vi "DNET Input.vi"(8 "stop":bool) -> (3 "DNET1":u32[](array[numeric]))   [LabVIEW 2011]
panel:
  in  "Slot":T1(ring)=enum."Dnet1"
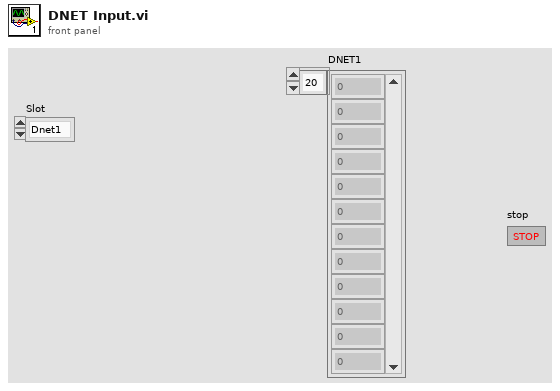
[diagram p1: front panel]
types:
  T1 = enum16{"NC1", "NC2", "Dnet1", "Dnet2", "Dnet3", "Ain1", "Ain2", "Aout1", "Din1", "Din2", "Dout1"}
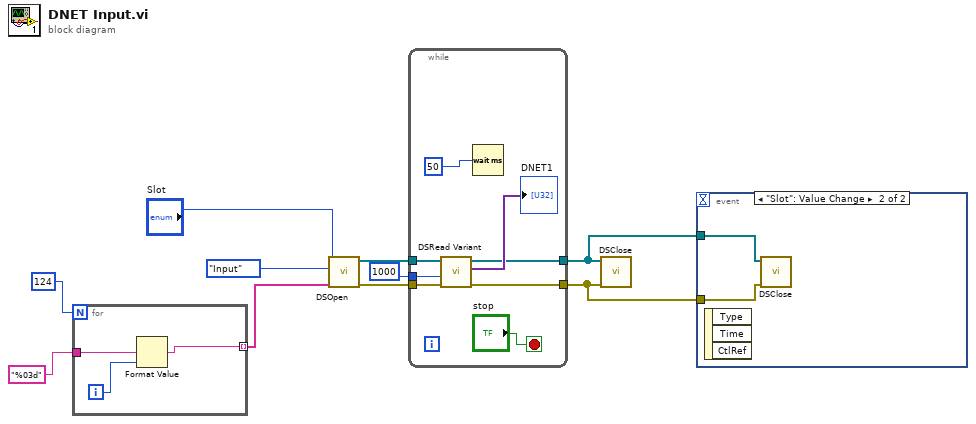
[diagram p0: block diagram]
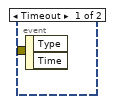
[diagram p2: hidden frame]
diagram:
  n1 = for {
    N: 124 -> [_]
    tunnel: "%03d" -> [w13]
    tunnel: [w12] -> w8 mode=indexing
    i -> [w11]
    n2 = Format Value(format string=w13, value (0)=w11) -> (output string=w12:string)  [unwired: 1 in]
  }
  n3 = call "DSOpen.vi"("Array"=w8, "I/O"=enum16{"Input", "Output"}."Input" ("Dnet I/O"), "Slot"="Slot") -> ("error Out"=w5:errorcluster[], "connection out"=w4:refnum<k13>[])  [unwired: 7 in]
  n4 = while {
    tunnel: w5 -> [w19]
    tunnel: w4 -> [w18]
    tunnel: 1000 -> [w17]
    tunnel: [w15] -> w2
    tunnel: [w14] -> w1
    stop <- "stop" stop-if-true
    n5 = call "DSRead Variant.vi"("error in"=w19, "ms timeout (10000)"=w17, "connection in"=w18) -> ("error out"=w14:errorcluster[], "data"=→"DNET1":variant[], "connection out"=w15:refnum<k13>[])  [unwired: 6 in]
    n6 = Wait (ms)(milliseconds to wait=u32 50) -> ()  [unwired: 1 out]
  }
  n7 = call "DSClose.vi"("error in (no error)"=w1, "connection id"=w2) -> ()  [unwired: 10 in]
  n8 = event shown="[1] \"Slot\": Value Change" {
    selector: _ -> [_ _]
    dyn-events: _ -> [_ _]
    timeout: _ -> [_ _]
    tunnel: w2 -> [_ w23]
    tunnel: w1 -> [_ w22]
    event Timeout {
      n9 = event-data() -> ()  [unwired: 1 in, 2 out]
    }
    event "Slot": Value Change {
      n10 = event-data() -> ()  [unwired: 1 in, 3 out]
      n11 = call "DSClose.vi"("error in (no error)"=w22, "connection id"=w23) -> ()  [unwired: 10 in]
    }
  }
